vi "Example from Pete.vi"   [LabVIEW 2020]
uses:
  99_Reference/LVMQTT-master/MQTT_Functions.lvlib
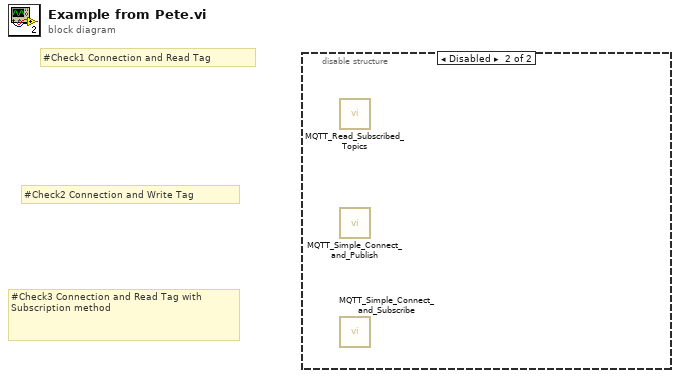
[diagram p0: block diagram]
diagram:
  # "#Check3 Connection and Read Tag with Subscription method"
  # "#Check2 Connection and Write Tag"
  # "#Check1 Connection and Read Tag"
  n1 = disable-structure shown="Disabled" {
    frame Enabled {
    }
    frame Disabled {
      n2 = call "MQTT_Read_Subscribed_Topics.vi"() -> ()  [unwired: 11 in, 1 out]
      n3 = call "MQTT_Simple_Connect_and_Publish.vi"() -> ()  [unwired: 12 in]
      n4 = call "MQTT_Simple_Connect_and_Subscribe.vi"() -> ()  [unwired: 12 in]
    }
  }
